vi "QueueToString.vi"(1 "QueueEnum":T1) -> (0 "String":string)   [LabVIEW 2012]
uses:
  QueueEnum.ctl
panel:
  in  "QueueArray":string[](array[string])=["cTankDrive", "cClimb", "cLauncherAngle", "cLauncherRPM", "cFirePneumatic"]
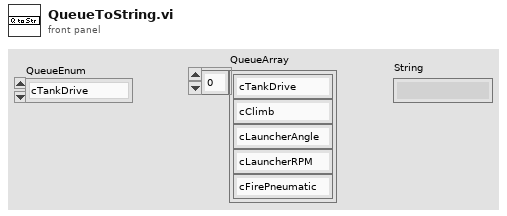
[diagram p1: front panel]
types:
  T1 = typedef "QueueEnum.ctl" = enum16{"cTankDrive", "cClimb", "cLauncherAngle", "cLauncherWheel", "cFirePneumatic"}
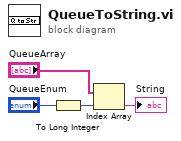
[diagram p0: block diagram]
diagram:
  n1 = To Long Integer(number="QueueEnum") -> (32bit integer=w2:i32)
  n2 = Index Array(array="QueueArray", index=w2) -> (element=→"String":string)
